vi "JPL Drivetrain Ramps and Curves.vi"(0 "Left Joystick Input":dbl(slide) scale=-10.0..10.0, 1 "Enable Curves":bool, 3 "Left Max Speed":dbl, 5 "Left Aux In":dbl, 7 "Delay Time (s)":dbl, 9 "Right Aux In":dbl, 11 "Right Joystick Input":dbl(slide) scale=-10.0..10.0, 12 "Enable Ramps":bool, 14 "Right Max Speed":dbl) -> (4 "Left Track Out":dbl, 15 "Right Track Out":dbl)   [LabVIEW 2015]
panel:
  out "Waveform Chart 2":cluster{"Slide":dbl, "Slide":dbl}(graph)
  out "Waveform Chart":cluster{"Slide":dbl, "Slide":dbl}(graph)
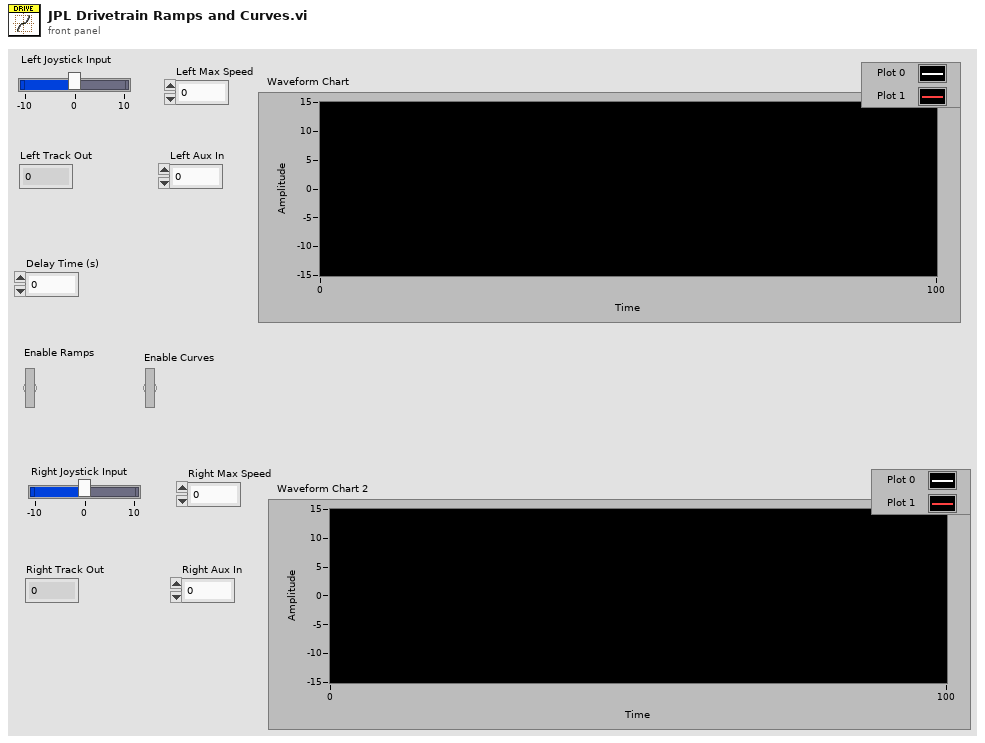
[diagram p1: front panel]
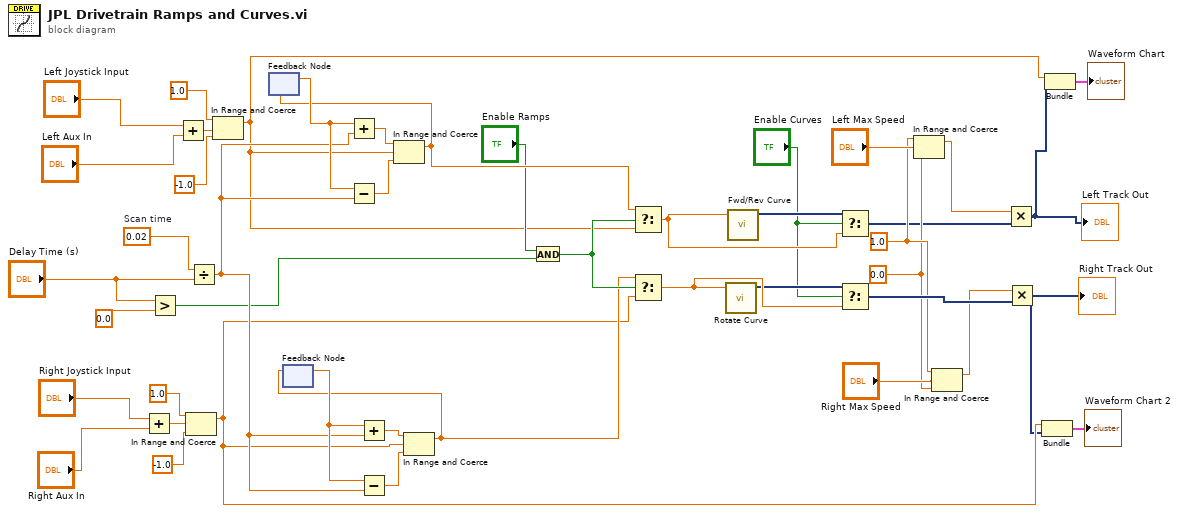
[diagram p0: block diagram]
diagram:
  w19 = 0.0
  w20 = 1.0
  w35 = 0.02  # Scan time
  n1 = Add(x="Right Joystick Input", y="Right Aux In") -> (x+y=w13:dbl)
  n2 = Greater?(x="Delay Time (s)", y=0.0) -> (0:w31:bool)
  n3 = Add(x="Left Joystick Input", y="Left Aux In") -> (x+y=w15:dbl)
  n4 = In Range and Coerce(upper limit=1.0, x=w13, lower limit=-1.0) -> (coerced(x)=w12:dbl)  [unwired: 1 out]
  n5 = Divide(x=w35, y="Delay Time (s)") -> (x/y=w34:dbl)
  n6 = In Range and Coerce(upper limit=1.0, x=w15, lower limit=-1.0) -> (coerced(x)=w14:dbl)  [unwired: 1 out]
  n7 = feedback #1() -> (w41:dbl)  [unwired: 1 in]
  n8 = feedback #2() -> (w37:dbl)  [unwired: 1 in]
  n9 = Add(x=w41, y=w34) -> (x+y=w44:dbl)
  n10 = Subtract(x=w41, y=w34) -> (x-y=w43:dbl)
  n11 = Add(x=w37, y=w34) -> (x+y=w40:dbl)
  n12 = Subtract(x=w37, y=w34) -> (x-y=w39:dbl)
  n13 = In Range and Coerce(upper limit=w44, x=w14, lower limit=w43) -> (coerced(x)=w36:dbl)  [unwired: 1 out]
  n14 = feedback-in #1(w36) -> ()
  n15 = In Range and Coerce(upper limit=w40, x=w12, lower limit=w39) -> (coerced(x)=w30:dbl)  [unwired: 1 out]
  n16 = feedback-in #2(w30) -> ()
  n17 = And(x="Enable Ramps", y=w31) -> (x .and. y?=w33:bool)
  n18 = Select(t=w36, s=w33, f=w14) -> (s? t:f=w29:dbl)
  n19 = Select(t=w30, s=w33, f=w12) -> (s? t:f=w28:dbl)
  n20 = call "Rotate Curve"("Signals"=w28) -> ("Scaled Signals"=w27:dynamicdata)  [unwired: 9 in, 1 out]
  n21 = call "Fwd/Rev Curve"("Signals"=w29) -> ("Scaled Signals"=w26:dynamicdata)  [unwired: 9 in, 1 out]
  n22 = Select(t=w26, s="Enable Curves", f=w29) -> (s? t:f=w1:dynamicdata)
  n23 = Select(t=w27, s="Enable Curves", f=w28) -> (s? t:f=w24:dynamicdata)
  n24 = In Range and Coerce(upper limit=w20, x="Left Max Speed", lower limit=w19) -> (coerced(x)=w22:dbl)  [unwired: 1 out]
  n25 = In Range and Coerce(upper limit=w20, x="Right Max Speed", lower limit=w19) -> (coerced(x)=w18:dbl)  [unwired: 1 out]
  n26 = Multiply(x=w22, y=w1) -> (x*y=w2:dynamicdata)
  "Left Track Out" <- w2
  n27 = Multiply(x=w18, y=w24) -> (x*y=w3:dynamicdata)
  "Right Track Out" <- w3
  n28 = Bundle(w12, w3) -> (→"Waveform Chart 2":cluster{dbl, dynamicdata})  [unwired: 1 in]
  n29 = Bundle(w14, w2) -> (→"Waveform Chart":cluster{dbl, dynamicdata})  [unwired: 1 in]
